vi "Anlagen-Grenzwerte SysLog.vi"(11 "NewVal":T1 {"Heizleitung zu FT-IR:"."Abschalt-Max" format="%#_5g"; "Heizleitung zu FT-IR:"."Abschalt-Min" format="%#_5g"; "Heizleitung zu FT-IR:"."Warn-Max" format="%#_5g"; "Heizleitung zu FT-IR:"."Warn-Min" format="%#_5g"; "Heizleitung zu FT-IR:"."Sollwert" format="%#_5g"; "Heizleitung zu FT-IR:"."Regler" items=["inaktiv", "aktiv"]; "Druck Kalter Block:"."Abschalt-Max" format="%#_5g"; "Druck Kalter Block:"."Abschalt-Min" format="%#_5g"; "Druck Kalter Block:"."Warn-Max" format="%#_5g"; "Druck Kalter Block:"."Warn-Min" format="%#_5g"; "Druck Kalter Block:"."Sollwert" format="%#_5g"; "Druck Kalter Block:"."Regler" items=["inaktiv", "aktiv"]; "Durchfluss CalGas:"."Abschalt-Max" format="%#_5g"; "Durchfluss CalGas:"."Abschalt-Min" format="%#_5g"; "Durchfluss CalGas:"."Warn-Max" format="%#_5g"; "Durchfluss CalGas:"."Warn-Min" format="%#_5g"; "Durchfluss CalGas:"."Sollwert" format="%#_5g"; "Durchfluss CalGas:"."Regler" items=["inaktiv", "aktiv"]; "Heizleitung Extern SP2:"."Abschalt-Max" format="%#_5g"; "Heizleitung Extern SP2:"."Abschalt-Min" format="%#_5g"; "Heizleitung Extern SP2:"."Warn-Max" format="%#_5g"; "Heizleitung Extern SP2:"."Warn-Min" format="%#_5g"; "Heizleitung Extern SP2:"."Sollwert" format="%#_5g"; "Heizleitung Extern SP2:"."Regler" items=["inaktiv", "aktiv"]; "Gaskühler:"."Abschalt-Max" format="%#_5g"; "Gaskühler:"."Abschalt-Min" format="%#_5g"; "Gaskühler:"."Warn-Max" format="%#_5g"; "Gaskühler:"."Warn-Min" format="%#_5g"; "Gaskühler:"."Sollwert" format="%#_5g"; "Gaskühler:"."Regler" items=["inaktiv", "aktiv"]; "Heizleitung Extern SP1:"."Abschalt-Max" format="%#_5g"; "Heizleitung Extern SP1:"."Abschalt-Min" format="%#_5g"; "Heizleitung Extern SP1:"."Warn-Max" format="%#_5g"; "Heizleitung Extern SP1:"."Warn-Min" format="%#_5g"; "Heizleitung Extern SP1:"."Sollwert" format="%#_5g"; "Heizleitung Extern SP1:"."Regler" items=["inaktiv", "aktiv"]; "Schaltschranktemperatur:"."Abschalt-Max" format="%#_5g"; "Schaltschranktemperatur:"."Abschalt-Min" format="%#_5g"; "Schaltschranktemperatur:"."Warn-Max" format="%#_5g"; "Schaltschranktemperatur:"."Warn-Min" format="%#_5g"; "Schaltschranktemperatur:"."Sollwert" format="%#_5g"; "Schaltschranktemperatur:"."Regler" items=["inaktiv", "aktiv"]; "FT-IR Heizung Messzelle:"."Abschalt-Max" format="%#_5g"; "FT-IR Heizung Messzelle:"."Abschalt-Min" format="%#_5g"; "FT-IR Heizung Messzelle:"."Warn-Max" format="%#_5g"; "FT-IR Heizung Messzelle:"."Warn-Min" format="%#_5g"; "FT-IR Heizung Messzelle:"."Sollwert" format="%#_5g"; "FT-IR Heizung Messzelle:"."Regler" items=["inaktiv", "aktiv"]; "Heizung Pumpe:"."Abschalt-Max" format="%#_5g"; "Heizung Pumpe:"."Abschalt-Min" format="%#_5g"; "Heizung Pumpe:"."Warn-Max" format="%#_5g"; "Heizung Pumpe:"."Warn-Min" format="%#_5g"; "Heizung Pumpe:"."Sollwert" format="%#_5g"; "Heizung Pumpe:"."Regler" items=["inaktiv", "aktiv"]; "Heizung Filterblock:"."Abschalt-Max" format="%#_5g"; "Heizung Filterblock:"."Abschalt-Min" format="%#_5g"; "Heizung Filterblock:"."Warn-Max" format="%#_5g"; "Heizung Filterblock:"."Warn-Min" format="%#_5g"; "Heizung Filterblock:"."Sollwert" format="%#_5g"; "Heizung Filterblock:"."Regler" items=["inaktiv", "aktiv"]; "Heizleitungen intern:"."Abschalt-Max" format="%#_5g"; "Heizleitungen intern:"."Abschalt-Min" format="%#_5g"; "Heizleitungen intern:"."Warn-Max" format="%#_5g"; "Heizleitungen intern:"."Warn-Min" format="%#_5g"; "Heizleitungen intern:"."Sollwert" format="%#_5g"; "Heizleitungen intern:"."Regler" items=["inaktiv", "aktiv"]; "Druck Ausgang:"."Abschalt-Max" format="%#_5g"; "Druck Ausgang:"."Abschalt-Min" format="%#_5g"; "Druck Ausgang:"."Warn-Max" format="%#_5g"; "Druck Ausgang:"."Warn-Min" format="%#_5g"; "Druck Ausgang:"."Sollwert" format="%#_5g"; "Druck Ausgang:"."Regler" items=["inaktiv", "aktiv"]; "Durchfluss FT-IR:"."Abschalt-Max" format="%#_5g"; "Durchfluss FT-IR:"."Abschalt-Min" format="%#_5g"; "Durchfluss FT-IR:"."Warn-Max" format="%#_5g"; "Durchfluss FT-IR:"."Warn-Min" format="%#_5g"; "Durchfluss FT-IR:"."Sollwert" format="%#_5g"; "Durchfluss FT-IR:"."Regler" items=["inaktiv", "aktiv"]; "Eingangsdruck FT-IR:"."Abschalt-Max" format="%#_5g"; "Eingangsdruck FT-IR:"."Abschalt-Min" format="%#_5g"; "Eingangsdruck FT-IR:"."Warn-Max" format="%#_5g"; "Eingangsdruck FT-IR:"."Warn-Min" format="%#_5g"; "Eingangsdruck FT-IR:"."Sollwert" format="%#_5g"; "Eingangsdruck FT-IR:"."Regler" items=["inaktiv", "aktiv"]}) -> (3 "NewVal out":T1 {"Heizleitung zu FT-IR:"."Abschalt-Max" format="%#_5g"; "Heizleitung zu FT-IR:"."Abschalt-Min" format="%#_5g"; "Heizleitung zu FT-IR:"."Warn-Max" format="%#_5g"; "Heizleitung zu FT-IR:"."Warn-Min" format="%#_5g"; "Heizleitung zu FT-IR:"."Sollwert" format="%#_5g"; "Heizleitung zu FT-IR:"."Regler" items=["inaktiv", "aktiv"]; "Druck Kalter Block:"."Abschalt-Max" format="%#_5g"; "Druck Kalter Block:"."Abschalt-Min" format="%#_5g"; "Druck Kalter Block:"."Warn-Max" format="%#_5g"; "Druck Kalter Block:"."Warn-Min" format="%#_5g"; "Druck Kalter Block:"."Sollwert" format="%#_5g"; "Druck Kalter Block:"."Regler" items=["inaktiv", "aktiv"]; "Durchfluss CalGas:"."Abschalt-Max" format="%#_5g"; "Durchfluss CalGas:"."Abschalt-Min" format="%#_5g"; "Durchfluss CalGas:"."Warn-Max" format="%#_5g"; "Durchfluss CalGas:"."Warn-Min" format="%#_5g"; "Durchfluss CalGas:"."Sollwert" format="%#_5g"; "Durchfluss CalGas:"."Regler" items=["inaktiv", "aktiv"]; "Heizleitung Extern SP2:"."Abschalt-Max" format="%#_5g"; "Heizleitung Extern SP2:"."Abschalt-Min" format="%#_5g"; "Heizleitung Extern SP2:"."Warn-Max" format="%#_5g"; "Heizleitung Extern SP2:"."Warn-Min" format="%#_5g"; "Heizleitung Extern SP2:"."Sollwert" format="%#_5g"; "Heizleitung Extern SP2:"."Regler" items=["inaktiv", "aktiv"]; "Gaskühler:"."Abschalt-Max" format="%#_5g"; "Gaskühler:"."Abschalt-Min" format="%#_5g"; "Gaskühler:"."Warn-Max" format="%#_5g"; "Gaskühler:"."Warn-Min" format="%#_5g"; "Gaskühler:"."Sollwert" format="%#_5g"; "Gaskühler:"."Regler" items=["inaktiv", "aktiv"]; "Heizleitung Extern SP1:"."Abschalt-Max" format="%#_5g"; "Heizleitung Extern SP1:"."Abschalt-Min" format="%#_5g"; "Heizleitung Extern SP1:"."Warn-Max" format="%#_5g"; "Heizleitung Extern SP1:"."Warn-Min" format="%#_5g"; "Heizleitung Extern SP1:"."Sollwert" format="%#_5g"; "Heizleitung Extern SP1:"."Regler" items=["inaktiv", "aktiv"]; "Schaltschranktemperatur:"."Abschalt-Max" format="%#_5g"; "Schaltschranktemperatur:"."Abschalt-Min" format="%#_5g"; "Schaltschranktemperatur:"."Warn-Max" format="%#_5g"; "Schaltschranktemperatur:"."Warn-Min" format="%#_5g"; "Schaltschranktemperatur:"."Sollwert" format="%#_5g"; "Schaltschranktemperatur:"."Regler" items=["inaktiv", "aktiv"]; "FT-IR Heizung Messzelle:"."Abschalt-Max" format="%#_5g"; "FT-IR Heizung Messzelle:"."Abschalt-Min" format="%#_5g"; "FT-IR Heizung Messzelle:"."Warn-Max" format="%#_5g"; "FT-IR Heizung Messzelle:"."Warn-Min" format="%#_5g"; "FT-IR Heizung Messzelle:"."Sollwert" format="%#_5g"; "FT-IR Heizung Messzelle:"."Regler" items=["inaktiv", "aktiv"]; "Heizung Pumpe:"."Abschalt-Max" format="%#_5g"; "Heizung Pumpe:"."Abschalt-Min" format="%#_5g"; "Heizung Pumpe:"."Warn-Max" format="%#_5g"; "Heizung Pumpe:"."Warn-Min" format="%#_5g"; "Heizung Pumpe:"."Sollwert" format="%#_5g"; "Heizung Pumpe:"."Regler" items=["inaktiv", "aktiv"]; "Heizung Filterblock:"."Abschalt-Max" format="%#_5g"; "Heizung Filterblock:"."Abschalt-Min" format="%#_5g"; "Heizung Filterblock:"."Warn-Max" format="%#_5g"; "Heizung Filterblock:"."Warn-Min" format="%#_5g"; "Heizung Filterblock:"."Sollwert" format="%#_5g"; "Heizung Filterblock:"."Regler" items=["inaktiv", "aktiv"]; "Heizleitungen intern:"."Abschalt-Max" format="%#_5g"; "Heizleitungen intern:"."Abschalt-Min" format="%#_5g"; "Heizleitungen intern:"."Warn-Max" format="%#_5g"; "Heizleitungen intern:"."Warn-Min" format="%#_5g"; "Heizleitungen intern:"."Sollwert" format="%#_5g"; "Heizleitungen intern:"."Regler" items=["inaktiv", "aktiv"]; "Druck Ausgang:"."Abschalt-Max" format="%#_5g"; "Druck Ausgang:"."Abschalt-Min" format="%#_5g"; "Druck Ausgang:"."Warn-Max" format="%#_5g"; "Druck Ausgang:"."Warn-Min" format="%#_5g"; "Druck Ausgang:"."Sollwert" format="%#_5g"; "Druck Ausgang:"."Regler" items=["inaktiv", "aktiv"]; "Durchfluss FT-IR:"."Abschalt-Max" format="%#_5g"; "Durchfluss FT-IR:"."Abschalt-Min" format="%#_5g"; "Durchfluss FT-IR:"."Warn-Max" format="%#_5g"; "Durchfluss FT-IR:"."Warn-Min" format="%#_5g"; "Durchfluss FT-IR:"."Sollwert" format="%#_5g"; "Durchfluss FT-IR:"."Regler" items=["inaktiv", "aktiv"]; "Eingangsdruck FT-IR:"."Abschalt-Max" format="%#_5g"; "Eingangsdruck FT-IR:"."Abschalt-Min" format="%#_5g"; "Eingangsdruck FT-IR:"."Warn-Max" format="%#_5g"; "Eingangsdruck FT-IR:"."Warn-Min" format="%#_5g"; "Eingangsdruck FT-IR:"."Sollwert" format="%#_5g"; "Eingangsdruck FT-IR:"."Regler" items=["inaktiv", "aktiv"]})   [LabVIEW 2020, in "Anlagengrenzwerte.lvlib"]
uses:
  Anlagengrenzwerte.lvlib
  Anlagen-Grenzwerte Anzeige.ctl
  Anlagen-Parameter Anzeige.ctl
  FGV Anlagengrenzwerte Aktionen.ctl
panel:
  # "°C"
  # "°C"
  # "°C"
  # "mbar"
  # "mbar"
  # "mbar"
  # "l/min"
  # "l/min"
  # "l/min"
  # "°C"
  # "°C"
  # "°C"
  # "°C"
  # "°C"
  # "°C"
  # "°C"
  # "°C"
  # "°C"
  # "°C"
  # "°C"
  # "°C"
  # "°C"
  # "°C"
  # "°C"
  # "°C"
  # "°C"
  # "°C"
  # "°C"
  # "°C"
  # "°C"
  # "°C"
  # "°C"
  # "°C"
  # "mbar"
  # "mbar"
  # "mbar"
  # "l/min"
  # "l/min"
  # "l/min"
  # "atm"
  # "atm"
  # "atm"
  # "°C"
  # "°C"
  # "°C"
  # "mbar"
  # "mbar"
  # "mbar"
  # "l/min"
  # "l/min"
  # "l/min"
  # "°C"
  # "°C"
  # "°C"
  # "°C"
  # "°C"
  # "°C"
  # "°C"
  # "°C"
  # "°C"
  # "°C"
  # "°C"
  # "°C"
  # "°C"
  # "°C"
  # "°C"
  # "°C"
  # "°C"
  # "°C"
  # "°C"
  # "°C"
  # "°C"
  # "°C"
  # "°C"
  # "°C"
  # "mbar"
  # "mbar"
  # "mbar"
  # "l/min"
  # "l/min"
  # "l/min"
  # "atm"
  # "atm"
  # "atm"
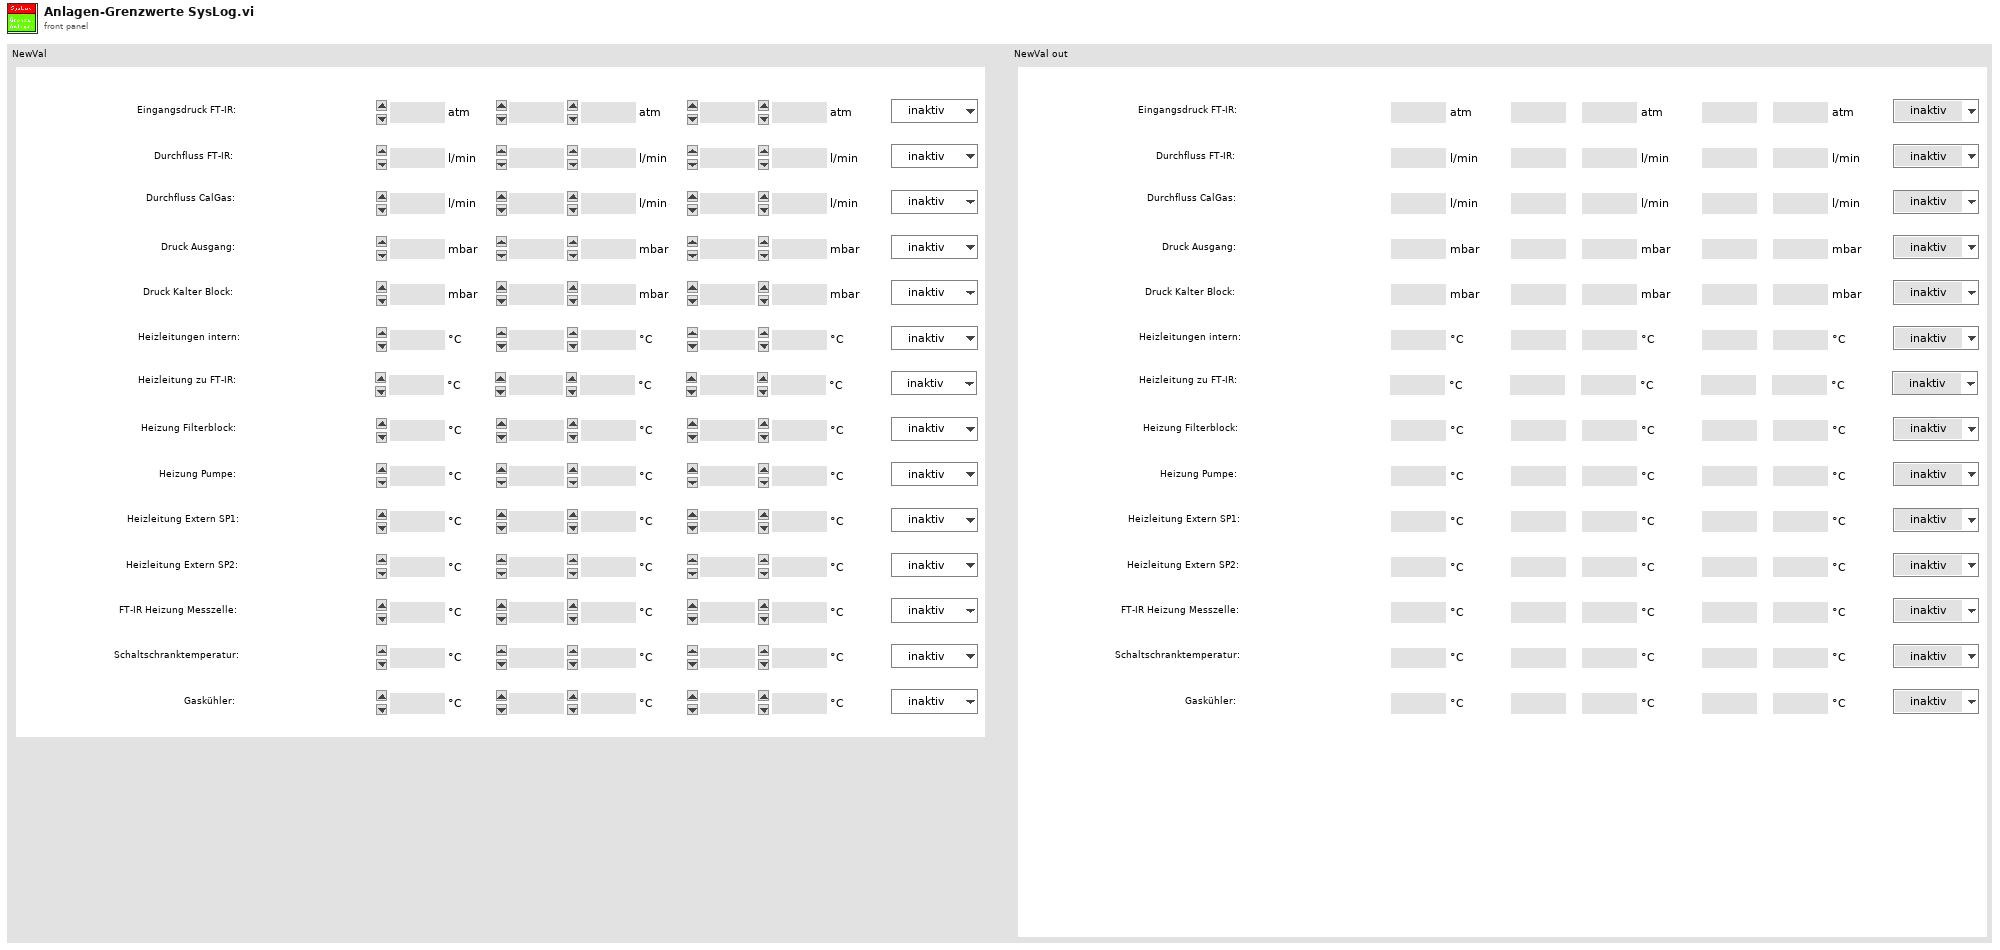
[diagram p1: front panel]
types:
  T1 = typedef "Anlagengrenzwerte.lvlib/Anlagen-Grenzwerte Anzeige.ctl" = cluster{"Eingangsdruck FT-IR:":T2, "Durchfluss FT-IR:":T2, "Durchfluss CalGas:":T2, "Druck Ausgang:":T2, "Druck Kalter Block:":T2, "Heizleitungen intern:":T2, "Heizleitung zu FT-IR:":T2, "Heizung Filterblock:":T2, "Heizung Pumpe:":T2, "Heizleitung Extern SP1:":T2, "Heizleitung Extern SP2:":T2, "FT-IR Heizung Messzelle:":T2, "Schaltschranktemperatur:":T2, "Gaskühler:":T2}
  T2 = typedef "Anlagengrenzwerte.lvlib/Anlagen-Parameter Anzeige.ctl" = cluster{"Sollwert":sgl, "Warn-Min":sgl, "Warn-Max":sgl, "Abschalt-Min":sgl, "Abschalt-Max":sgl, "Regler":u16}
  T3 = typedef "Anlagengrenzwerte.lvlib/FGV Anlagengrenzwerte Aktionen.ctl" = enum16{"Lesen", "Grenzwerte schreiben"}
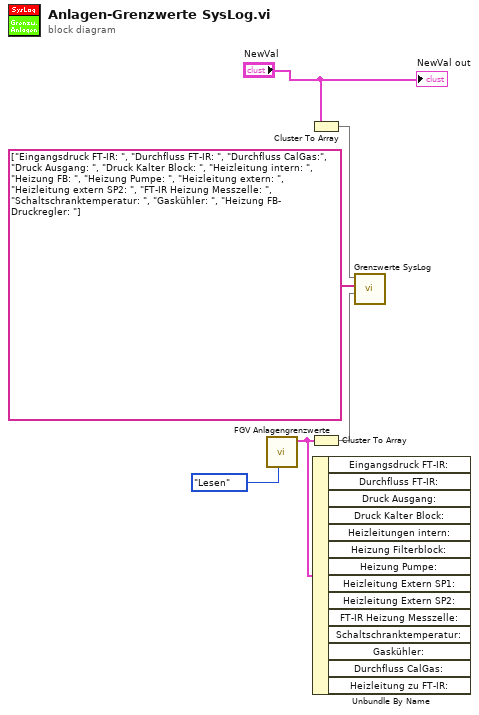
[diagram p0: block diagram]
diagram:
  n1 = call "FGV Anlagengrenzwerte.vi"("Aktion"=FGV_Anlagengrenzwerte_Aktionen."Lesen") -> ("Anlagen-Grenzwerte Anzeige"=w5:T1)  [unwired: 1 in, 9 out]
  n2 = Cluster To Array(cluster="NewVal") -> (array=w1:T2[])
  n3 = Cluster To Array(cluster=w5) -> (array=w2:T2[])
  n4 = Unbundle By Name(w5) -> ()  [unwired: 14 out]
  n5 = call "Grenzwerte SysLog.vi"("Anlagen-Grenzwerte Anzeige"=w2, "Fehlermeldung"=string[] ["Eingangsdruck FT-IR: ", "Durchfluss FT-IR: ", "Durchfluss CalGas:", "Druck Ausgang: ", "Druck Kalter Block: ", "Heizleitung intern: ", "Heizung FB: ", "Heizung Pumpe: ", "Heizleitung extern: ", "Heizleitung extern SP2: ", "FT-IR Heizung Messzelle: ", "Schaltschranktemperatur: ", "Gaskühler: ", "Heizung FB- Druckregler: "], "NewVal"=w1) -> ()  [unwired: 9 in]
  "NewVal out" <- "NewVal"
